vi "Load Set.vi"() -> (2 "Set":T1[](array[typedef])=[{"Clef"=enum."Treble", "Note Number"=12}, {"Clef"=enum."Treble", "Note Number"=0}, {"Clef"=enum."Bass", "Note Number"=0}, {"Clef"=enum."Bass", "Note Number"=-12}])   [LabVIEW 2014]
uses:
  Type Defs/Note Definition.ctl
  Type Defs/Clef.ctl
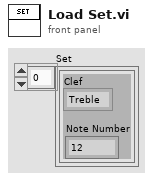
[diagram p1: front panel]
types:
  T1 = typedef "Note Definition.ctl" = cluster{"Clef":T2, "Note Number":i16}
  T2 = typedef "Clef.ctl" = enum16{"Treble", "Bass"}
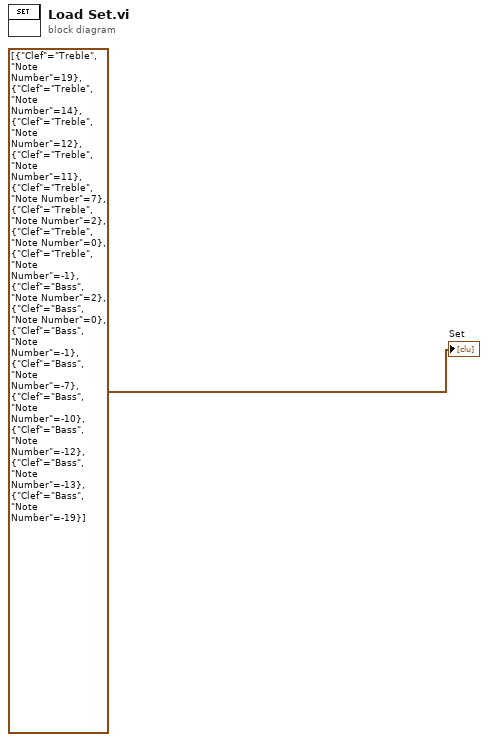
[diagram p0: block diagram]
diagram:
  "Set" <- T1[] [{"Clef"=enum."Treble", "Note Number"=19}, {"Clef"=enum."Treble", "Note Number"=14}, {"Clef"=enum."Treble", "Note Number"=12}, {"Clef"=enum."Treble", "Note Number"=11}, {"Clef"=enum."Treble", "Note Number"=7}, {"Clef"=enum."Treble", "Note Number"=2}, {"Clef"=enum."Treble", "Note Number"=0}, {"Clef"=enum."Treble", "Note Number"=-1}, {"Clef"=enum."Bass", "Note Number"=2}, {"Clef"=enum."Bass", "Note Number"=0}, {"Clef"=enum."Bass", "Note Number"=-1}, {"Clef"=enum."Bass", "Note Number"=-7}, {"Clef"=enum."Bass", "Note Number"=-10}, {"Clef"=enum."Bass", "Note Number"=-12}, {"Clef"=enum."Bass", "Note Number"=-13}, {"Clef"=enum."Bass", "Note Number"=-19}]
